vi "AES - Example.vi"() -> ()   [LabVIEW 2013]
panel:
  out "encrypted string (hex)":string
  out "encrypted string (base 64)":string
  out "decrypted string":string
  in  "string to encrypt":string="I Love MoM!"
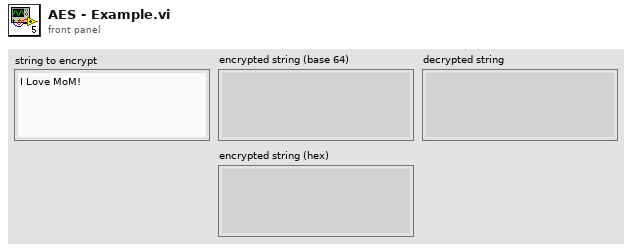
[diagram p1: front panel]
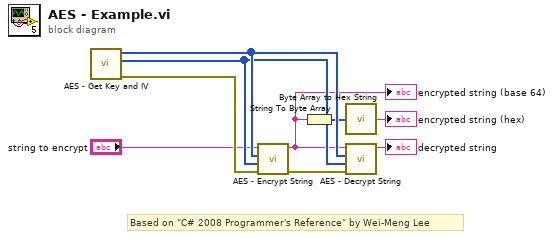
[diagram p0: block diagram]
diagram:
  # "Based on \"C# 2008 Programmer's Reference\" by Wei-Meng Lee"
  n1 = call "AES - Get Key and IV.vi"() -> ("error out"=w9:errorcluster, "IV"=w6:u8[], "Key"=w7:u8[])  [unwired: 9 in]
  n2 = call "AES - Encrypt String.vi"("error in (no error)"=w9, "IV"=w6, "key"=w7, "string to encrypt"="string to encrypt") -> ("error out"=w8:errorcluster, "encrypted string"=w2:string)  [unwired: 6 in]
  "encrypted string (base 64)" <- w2
  n3 = String To Byte Array(string=w2) -> (unsigned byte array=w3:u8[])
  n4 = call "Byte Array to Hex String.vi"("bytes array"=w3) -> ("hex string"=→"encrypted string (hex)":string)
  n5 = call "AES - Decrypt String.vi"("error in (no error)"=w8, "IV"=w6, "key"=w7, "encrypted string"=w2) -> ("decrypted string"=→"decrypted string":string)  [unwired: 6 in, 1 out]
